vi "Get FPGA Device Info.vi"(8 "error in (no error)":errorcluster) -> (0 "error out":errorcluster, 2 "FPGA Devices":refnum<class "FPGA Device.lvclass">[](array[class]))   [LabVIEW 2016, in "FPGA RM Engine API.lvlib"]
uses:
  FPGA RM Engine API.lvlib
  Shared/FPGA Configuration Classes/FPGA Device/FPGA Device.lvclass
  <vilib>/NI Veristand/Custom Device API/Custom Device Item Ref.ctl
  Shared/FPGA RM Shared API.lvlib
  <vilib>/NI VeriStand/Custom Device API/Custom Device API.lvlib
panel:
  out "Item Ref out":T1 format="%.0x"
  in  "Item Ref in":T1 format="%.0x"
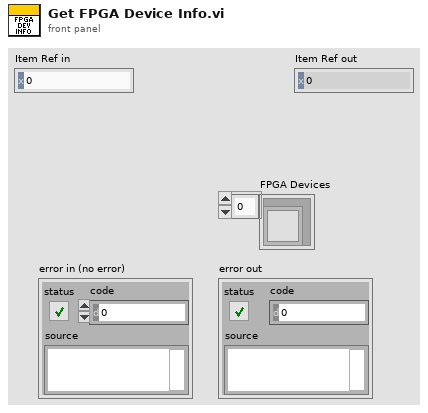
[diagram p1: front panel]
types:
  T1 = typedef "Custom Device API.lvlib/Custom Device Item Ref.ctl" = u64
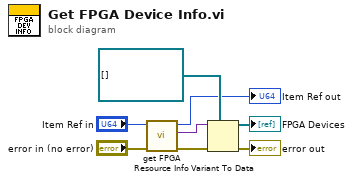
[diagram p0: block diagram]
diagram:
  n1 = call "get FPGA Resource Info.vi"("error in (no error)"="error in (no error)", "CD Ref in"="Item Ref in") -> ("error out"=w4:errorcluster, "Value"=w2:variant, "Item Ref out"=→"Item Ref out":T1)  [unwired: 7 in]
  n2 = Variant To Data(error in=w4, type=refnum<class "FPGA Device.lvclass">[] [] ("Array"), Variant=w2) -> (data=→"FPGA Devices":refnum<class "FPGA Device.lvclass">[], error out=→"error out":errorcluster)
